vi "ExSubInitNOpenCam_new.vi"(0 "error in (no error)":errorcluster) -> (1 "Camera Handle":u32, 3 "error out":errorcluster)   [LabVIEW 2014]
uses:
  Public/Documents/SIToolkit/LabVIEW/Examples2014_6_0_2_9/Fast Examples/Open-Close Hardware/CamHandle.vi
panel:
  # "ExSubInitNOpenCam:\nThis is a SubVI which initializes the SITK(tm) toolkit\nand opens a camera. If successful it returns a \ncamera handle."
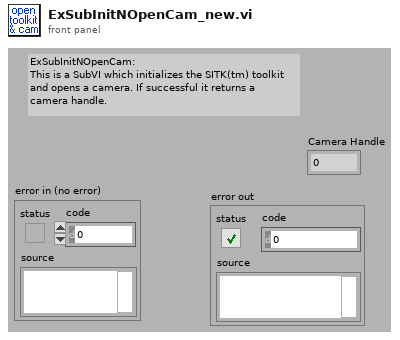
[diagram p1: front panel]
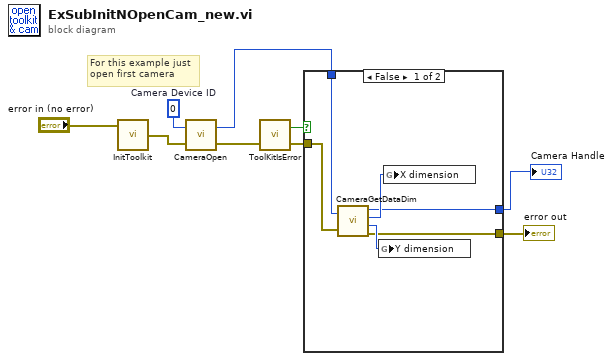
[diagram p0: block diagram]
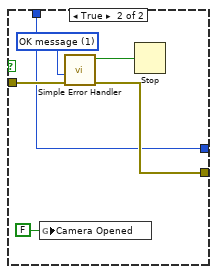
[diagram p2: hidden frame]
diagram:
  w5 = u32 0  # Camera Device ID
  # "For this example just\nopen first camera"
  n1 = call <userlib>:"InitToolkit.vi"("error in"="error in (no error)") -> ("error out"=w9:errorcluster)
  n2 = call <userlib>:"CameraOpen.vi"("error in"=w9, "Camera Device ID"=w5) -> ("error out"=w8:errorcluster, "Camera Handle"=w4:u32)
  n3 = call <userlib>:"ToolKitIsError.vi"("error in"=w8) -> ("error out"=w6:errorcluster, "Error Flag"=w7:bool)  [unwired: 1 in]
  n4 = case shown="False" w7 {
    tunnel: w6 -> [w12 w21]
    tunnel: w4 -> [w13 w17]
    tunnel: [w11 w18] -> w2
    tunnel: [w10 w17] -> w3
    frame False {
      n5 = call <userlib>:"CameraGetDataDim.vi"("Camera Handle"=w13, "error in"=w12) -> ("Camera Handle"=w10:u32, "Xdim"=w14:u32, "Ydim"=w15:u32, "error out"=w11:errorcluster)
      n6 = global write "CamHandle.vi" "Y dimension"(w15) -> ()
      n7 = global write "CamHandle.vi" "X dimension"(w14) -> ()
    }
    frame True {
      w19 = u16 1 items=["no dialog", "OK message", "continue or stop message"] ("type of dialog (OK msg:1)")
      n8 = global write "CamHandle.vi" "Camera Opened"(FALSE ("Camera Opened")) -> ()
      n9 = call <vilib>:"Simple Error Handler.vi"("type of dialog (OK msg:1)"=w19, "error in (no error)"=w21) -> ("error?"=w20:bool, "error out"=w18:errorcluster)  [unwired: 3 in, 3 out]
      n10 = Stop(stop? (T)=w20) -> ()
    }
  }
  "Camera Handle" <- w3
  "error out" <- w2
